vi "LoadFaceEncoding.vi"(8 "error in (no error)":errorcluster, 10 "encoding":dbl[](array[numeric]), 11 "FaceRecognition in":refnum<class "FaceRecognition.lvclass">) -> (0 "error out":errorcluster, 2 "LoadFaceEncoding":refnum<k24>, 3 "FaceRecognition out":refnum<class "FaceRecognition.lvclass">)   [LabVIEW 2020, in "FaceRecognitionDotNet.lvlib" / "FaceRecognition.lvclass"]
uses:
  FaceRecognition.lvclass
  dll/FaceRecognitionDotNet.dll
  FaceRecognition.lvclass/FaceRecognition.ctl
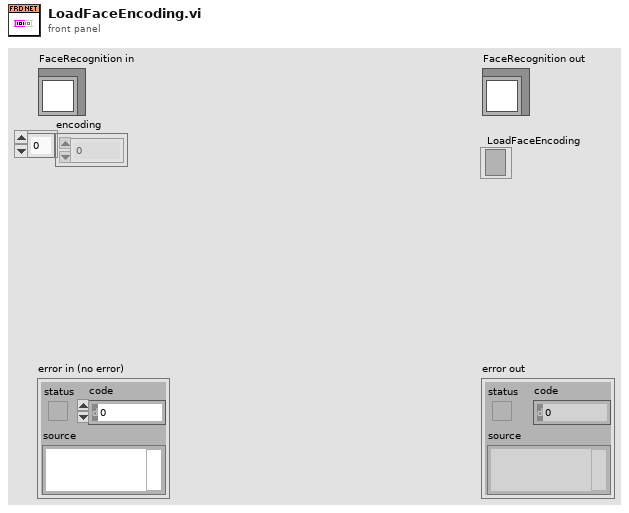
[diagram p1: front panel]
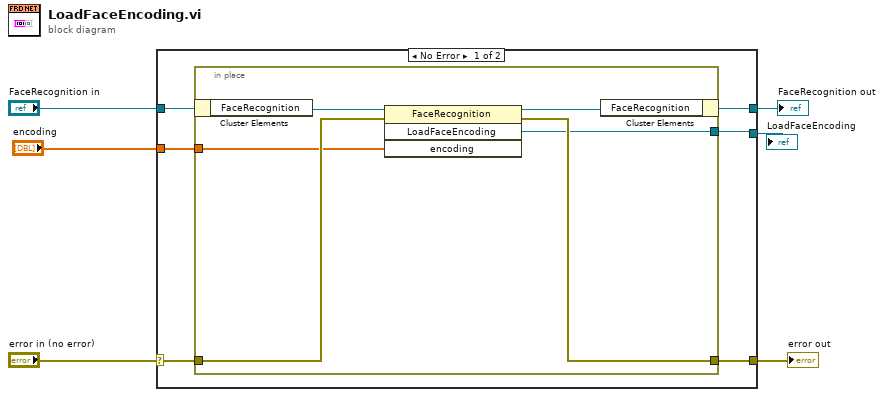
[diagram p0: block diagram]
diagram:
  n1 = case shown="No Error" "error in (no error)" {
    selector: "error in (no error)" -> [w10 w20]
    tunnel: [w9 w20] -> w5
    tunnel: [w11 w19] -> w3
    tunnel: "FaceRecognition in" -> [w12 w19]
    tunnel: [w8 _] -> w1
    tunnel: "encoding" -> [w7 _]
    frame No Error {
      n2 = in-place {
        in-place-border: w10 -> [w16]
        in-place-border: [w15] -> w9
        in-place-border: [w14] -> w8
        in-place-border: w7 -> [w13]
        n3 = in-place-cluster #1(w12) -> ("FaceRecognition"=w18:refnum<k24>)
        n4 = invoke class="FaceRecognition" method="LoadFaceEncoding"(reference=w18, error in=w16, "encoding"=w13) -> (reference out=w17:refnum<k24>, error out=w15:errorcluster, "LoadFaceEncoding"=w14:refnum<k24>)  [unwired: 1 in, 1 out]
        n5 = in-place-cluster #1("FaceRecognition"=w17) -> (w11:refnum<class "FaceRecognition.lvclass">)
      }
    }
    frame Error {
    }
  }
  "error out" <- w5
  "FaceRecognition out" <- w3
  "LoadFaceEncoding" <- w1
